vi "timming_array_to_digital_waveform.vi"(3 "delay array":dbl[](array[numeric]) format="%#_6e", 4 "resolution":i32=100) -> (0 "digital waveform":digitalwaveform(waveform)={"t0"=timestamp(0 s since 1904-01-01), "dt"=0.0, "Y"={"transitions"=[], "data"=[]}, "error"={"status"=FALSE, "code"=37421928, "source"=""}})   [LabVIEW 2011]
doc: "takes the timing info recieved from the DG645 Delay generator and transforms it into a digital waveform graph.\nMakes sure, all timings are setup in reference to t0!"
uses:
  <vilib>/Waveform/DWDTOps.llb/DWDT Boolean Array to Digital.vi
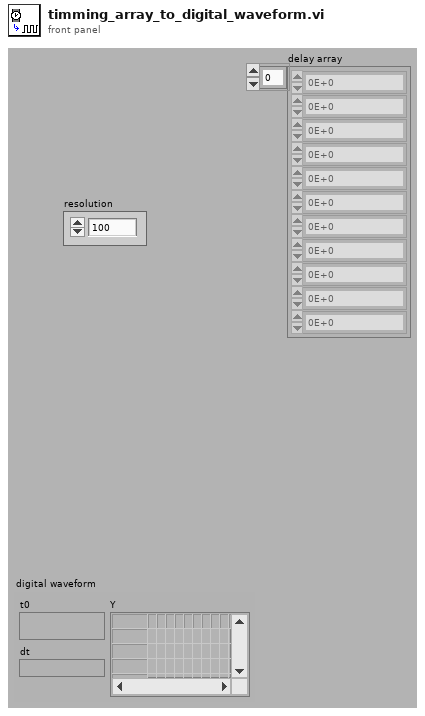
[diagram p1: front panel]
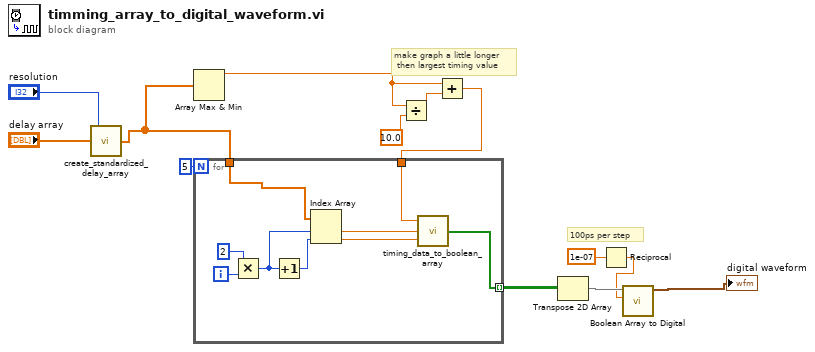
[diagram p0: block diagram]
diagram:
  # "100ps per step"
  # "make graph a little longer\n then largest timing value"
  n1 = call "create_standardized_delay_array.vi"("delay array"="delay array", "resolution"="resolution") -> ("standardize array"=w2:dbl[])  [unwired: 2 in, 1 out]
  n2 = Array Max & Min(array=w2) -> (max value=w5:dbl)  [unwired: 3 out]
  n3 = Divide(x=w5, y=10.0) -> (x/y=w9:dbl)
  n4 = Add(x=w5, y=w9) -> (x+y=w6:dbl)
  n5 = for {
    N: 5 -> [_]
    tunnel: [w20] -> w12 mode=indexing
    tunnel: w6 -> [w19]
    tunnel: w2 -> [w14]
    i -> [w22]
    n6 = Multiply(x=2, y=w22) -> (x*y=w15:i32)
    n7 = Increment(x=w15) -> (x+1=w18:i32)
    n8 = Index Array(array=w14, index #1=w15, index #2=w18) -> (element #1=w17:dbl, element #2=w16:dbl)
    n9 = call "timing_data_to_boolean_array.vi"("end time [us]"=w16, "start time [us]"=w17, "overall length [us]"=w19) -> ("boolean timing array"=w20:bool[])  [unwired: 1 in]
  }
  n10 = Transpose 2D Array(2D array=w12) -> (transposed array=w11:bool[][])
  n11 = Reciprocal(x=1e-07) -> (1/x=w7:dbl)
  n12 = call-poly <vilib>:"Boolean Array to Digital.vi"("sample rate"=w7, "boolean array"=w11) -> ("digital waveform"=→"digital waveform":digitalwaveform)  [unwired: 8 in, 1 out]
